vi "Patient_Heart_LabView.vi"() -> ()   [LabVIEW 2020]
panel:
  in  "VISA resource name":refnum<visa-resource-name>
  in  "Patient's Data":string[][](table)
  out "Temp":dbl(graph)
  out "Heart Rate BPM":dbl(graph)
  out "Temp":dbl(slide) scale=0.0..100.0
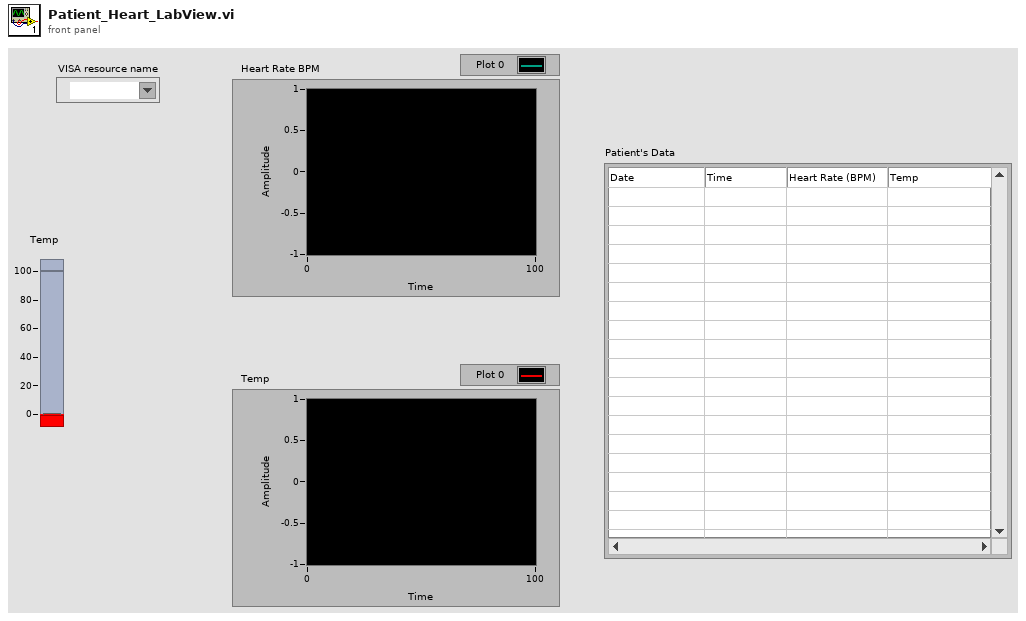
[diagram p1: front panel]
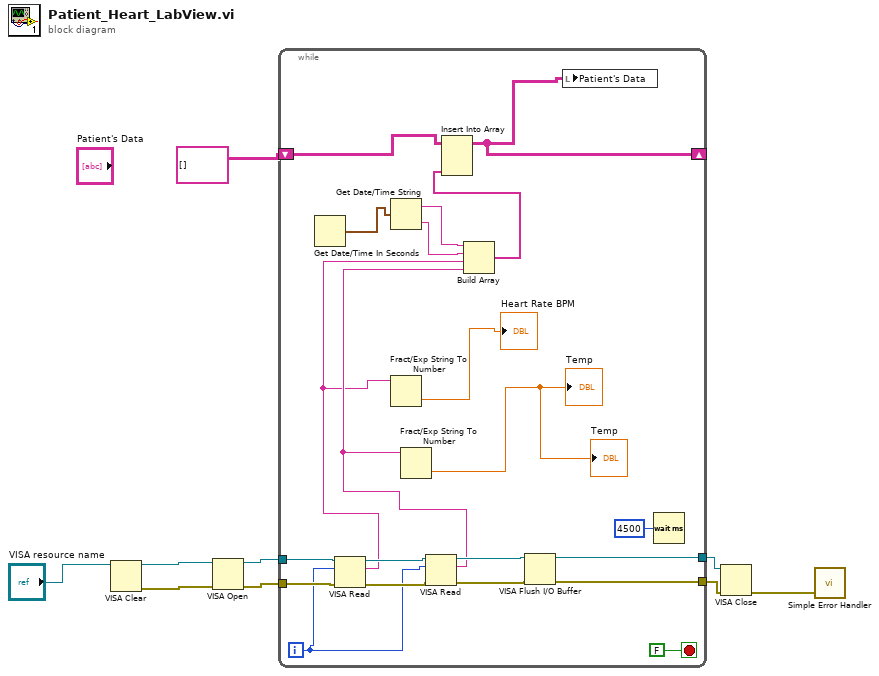
[diagram p0: block diagram]
diagram:
  n1 = VISA Clear(VISA resource name="VISA resource name") -> (VISA resource name out=w9:refnum<visa-resource-name>, error out=w8:errorcluster)  [unwired: 1 in]
  n2 = VISA Open(error in (no error)=w8, VISA resource name=w9) -> (VISA resource name=w7:refnum<visa-resource-name>, error out=w5:errorcluster)  [unwired: 3 in]
  n3 = while {
    tunnel: w7 -> [w30]
    tunnel: [w27] -> w6
    tunnel: w5 -> [w26]
    tunnel: [w23] -> w4
    shift-right: [w19] -> _
    shift-left: string[][] [] -> [w20]
    i -> [w22]
    stop <- FALSE stop-if-true
    n4 = Get Date/Time In Seconds() -> (seconds since 1Jan1904=w16:timestamp)
    n5 = VISA Read(VISA resource name=w30, byte count=w22, error in (no error)=w26) -> (VISA resource name out=w29:refnum<visa-resource-name>, read buffer=w12:string, error out=w25:errorcluster)  [unwired: 1 out]
    n6 = Get Date/Time String(seconds (now)=w16) -> (date string=w15:string, time string=w14:string)  [unwired: 2 in]
    n7 = Fract/Exp String To Number(string=w12) -> (number=→"Heart Rate BPM":dbl)  [unwired: 3 in, 1 out]
    n8 = VISA Read(VISA resource name=w29, byte count=w22, error in (no error)=w25) -> (VISA resource name out=w28:refnum<visa-resource-name>, read buffer=w13:string, error out=w24:errorcluster)  [unwired: 1 out]
    n9 = Fract/Exp String To Number(string=w13) -> (number=→"Temp" →"Temp":dbl)  [unwired: 3 in, 1 out]
    n10 = Build Array(w15, w14, w12, w13) -> (w11:string[])
    n11 = Insert Into Array(array=w20, new element=w11) -> (w19:string[][])  [unwired: 2 in]
    n12 = VISA Flush I/O Buffer(VISA resource name=w28, error in (no error)=w24) -> (VISA resource name out=w27:refnum<visa-resource-name>, error out=w23:errorcluster)  [unwired: 1 in]
    n13 = local write "Patient's Data"(w19) -> ()
    n14 = Wait (ms)(milliseconds to wait=u32 4500) -> ()  [unwired: 1 out]
  }
  n15 = VISA Close(VISA resource name=w6, error in (no error)=w4) -> (error out=w3:errorcluster)
  n16 = call <vilib>:"Simple Error Handler.vi"("error in (no error)"=w3) -> ()  [unwired: 4 in, 5 out]
